vi "Get Libraries in Project.vi"(0 "Project path":path, 11 "error in (no error)":errorcluster) -> (4 "Project exists?":bool, 6 "Library names":string[](array[string]), 15 "error out":errorcluster)   [LabVIEW 2021, in "Migrator.lvlib"]
uses:
  Migrator.lvlib
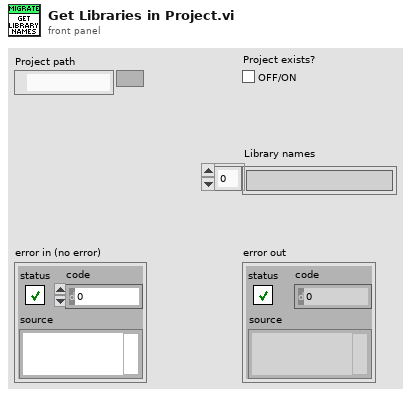
[diagram p1: front panel]
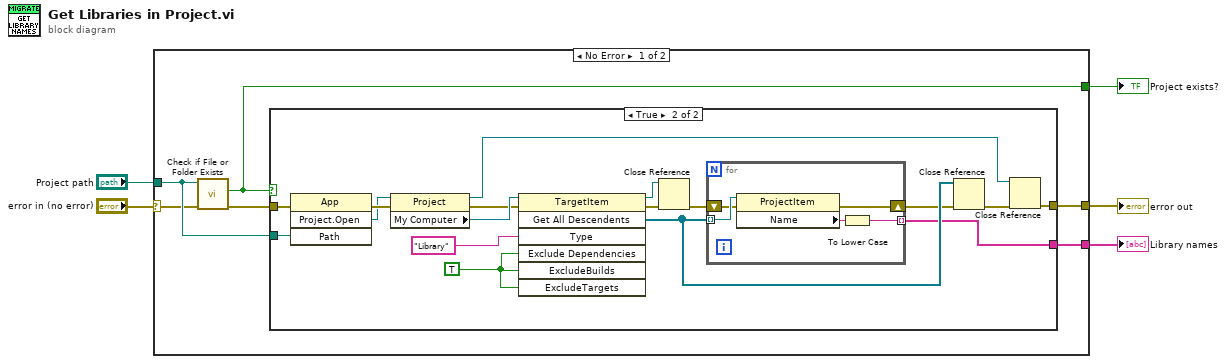
[diagram p0: block diagram]
diagram:
  n1 = case shown="No Error" "error in (no error)" {
    selector: "error in (no error)" -> [w9 w35]
    tunnel: "Project path" -> [w10 _]
    tunnel: [w11 w35] -> w3
    tunnel: [w7 _] -> w2
    tunnel: [w6 _] -> w1
    frame No Error {
      n2 = call <vilib>:"Check if File or Folder Exists.vi"("error in (no error)"=w9, "path"=w10) -> ("error out"=w8:errorcluster, "file or folder exists?"=w7:bool)  [unwired: 7 in, 1 out]
      n3 = case shown="True" w7 {
        tunnel: [w12 w20] -> w11
        tunnel: w10 -> [_ w23]
        tunnel: w8 -> [w12 w22]
        tunnel: [_ w13] -> w6
        frame False {
        }
        frame True {
          w17 = TRUE ("ExcludeDependencies")
          n4 = invoke class="App" method="Project.Open"(error in=w22, "Path"=w23) -> (error out=w24:errorcluster, "Project:Open"=w21:refnum<vi>)  [unwired: 2 in, 2 out]
          n5 = property class="Project"(reference=w21, error in=w24) -> (reference out=w19:refnum<vi>, error out=w28:errorcluster, "My Computer"=w29:refnum<vi>)
          n6 = invoke class="TargetItem" method="Get All Descendents"(reference=w29, error in=w28, "Type"="Library", "Exclude Dependencies"=w17, "ExcludeBuilds"=w17, "ExcludeTargets"=w17) -> (reference out=w26:refnum<vi>, error out=w27:errorcluster, "All Descendents"=w16:refnum<vi>[])  [unwired: 1 in, 4 out]
          n7 = Close Reference(reference=w26, error in (no error)=w27) -> (error out=w18:errorcluster)
          n8 = for {
            tunnel: w16 -> [w34] mode=indexing
            shift-right: [w32] -> w14
            shift-left: w18 -> [w33]
            tunnel: [w30] -> w13 mode=indexing
            n9 = property class="ProjectItem"(reference=w34, error in=w33) -> (error out=w32:errorcluster, "Name"=w31:string)  [unwired: 1 out]
            n10 = To Lower Case(string=w31) -> (all lower case string=w30:string)
          }
          n11 = Close Reference(reference=w16, error in (no error)=w14) -> (error out=w15:errorcluster)
          n12 = Close Reference(reference=w19, error in (no error)=w15) -> (error out=w20:errorcluster)
        }
      }
    }
    frame Error {
    }
  }
  "error out" <- w3
  "Project exists?" <- w2
  "Library names" <- w1
